vi "Baseline array.vi"(7 "Detected event (1D)":cluster{dbl[][]}[](array[cluster])) -> (3 "Baseline array":cluster{T1[]}[](array[cluster]))   [LabVIEW 2017]
uses:
  Baseline selection.ctl
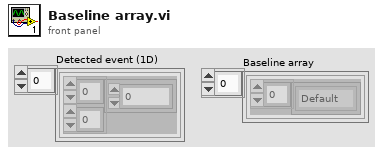
[diagram p1: front panel]
types:
  T1 = typedef "Baseline selection.ctl" = enum16{"Default", "Manual"}
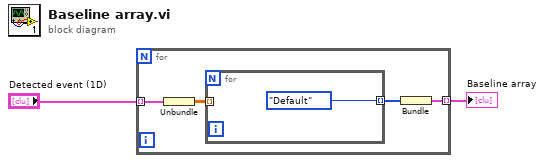
[diagram p0: block diagram]
diagram:
  n1 = for {
    tunnel: "Detected event (1D)" -> [w6] mode=indexing
    tunnel: [w3] -> w1 mode=indexing
    n2 = Unbundle(w6) -> (w5:dbl[][])
    n3 = for {
      tunnel: w5 -> [_] mode=indexing
      tunnel: [Baseline_selection."Default" ("Baseline selection")] -> w4 mode=indexing
    }
    n4 = Bundle(w4) -> (w3:cluster{T1[]})  [unwired: 1 in]
  }
  "Baseline array" <- w1
